vi "Process.vi"(0 "reg.notify host.go rcvd":bool, 1 "reg.reset":bool, 2 "reg.instruction fifo":refnum<k21>, 5 "reg.host read.go rcvd":bool, 7 "clock cross resources":T7, 9 "config.resources":T5, 11 "sync.resources":T6, 12 "time.resources":T3) -> (4 "reg.notify host.go":bool, 6 "reg.host read.data":T4)   [LabVIEW 2021]
doc: "The main process loop which sends instructions received from the host to its attached registers and returns register reads back to the host."
uses:
  Clock Cross Resources.ctl
  <instrlib>/niUsrpRio/Synchronization/v1/FPGA/Private/Resources.ctl
  <instrlib>/_niInstr/Register Bus/v1/FPGA/Public/Read Cmd Data.ctl
  <instrlib>/niUsrpRio/Time/v1/FPGA/Private/Time Resources.ctl
  <instrlib>/niUsrpRio/Time/v1/FPGA/Private/Future Event Resources.ctl
  <instrlib>/_niInstr/Register Bus/v1/FPGA/Public/Read Completion.ctl
  <instrlib>/_niInstr/Register Bus/v1/FPGA/Private/Mux/Read Completion Mux (2 inputs).vi
  <instrlib>/_niInstr/Register Bus/v1/FPGA/niInstr Register Bus v1 FPGA.lvlib
  <instrlib>/niUsrpRio/Synchronization/v1/FPGA/niUsrpRio Synchronization v1 FPGA.lvlib
  <instrlib>/niUsrpRio/Time/v1/FPGA/niUsrpRio Time v1 FPGA.lvlib
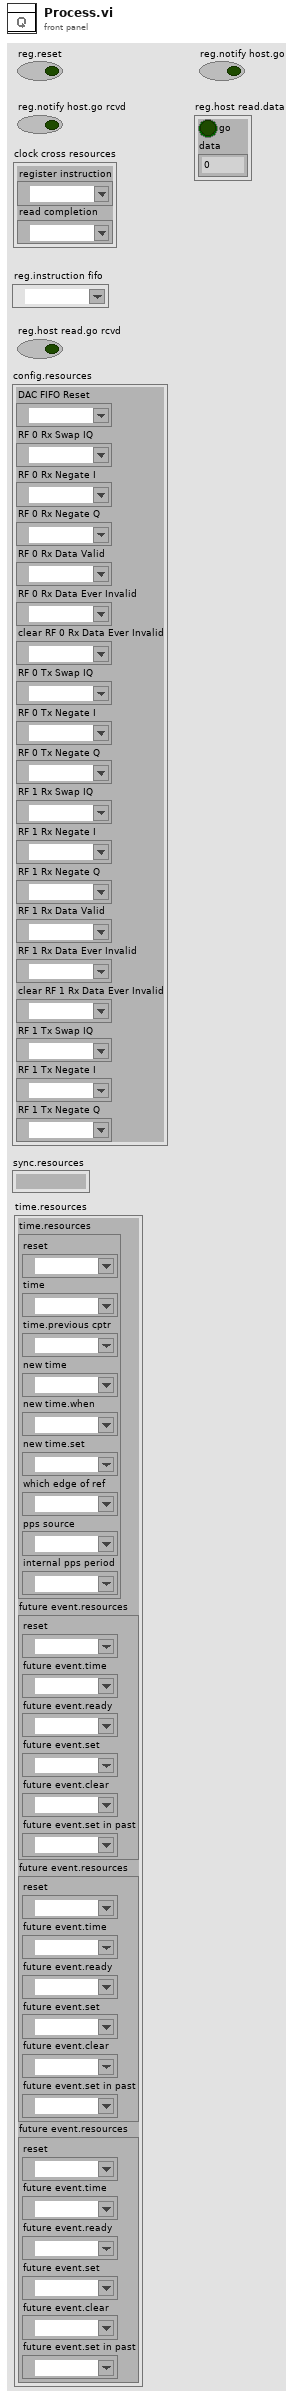
[diagram p1: front panel]
types:
  T1 = typedef "niUsrpRio Time v1 FPGA.lvlib/Time Resources.ctl" = cluster{"reset":refnum<k21>, "time":refnum<k21>, "time.previous cptr":refnum<k21>, "new time":refnum<k21>, "new time.when":refnum<k21>, "new time.set":refnum<k21>, "which edge of ref":refnum<k21>, "pps source":refnum<k21>, "internal pps period":refnum<k21>}
  T2 = typedef "niUsrpRio Time v1 FPGA.lvlib/Future Event Resources.ctl" = cluster{"reset":refnum<k21>, "future event.time":refnum<k21>, "future event.ready":refnum<k21>, "future event.set":refnum<k21>, "future event.clear":refnum<k21>, "future event.set in past":refnum<k21>}
  T3 = cluster{"time.resources":T1, "future event.resources":T2, "future event.resources":T2, "future event.resources":T2}
  T4 = typedef "niInstr Register Bus v1 FPGA.lvlib/Read Cmd Data.ctl" = cluster{"go":bool, "data":u32}
  T5 = cluster{"DAC FIFO Reset":refnum<k21>, "RF 0 Rx Swap IQ":refnum<k21>, "RF 0 Rx Negate I":refnum<k21>, "RF 0 Rx Negate Q":refnum<k21>, "RF 0 Rx Data Valid":refnum<k21>, "RF 0 Rx Data Ever Invalid":refnum<k21>, "clear RF 0 Rx Data Ever Invalid":refnum<k21>, "RF 0 Tx Swap IQ":refnum<k21>, "RF 0 Tx Negate I":refnum<k21>, "RF 0 Tx Negate Q":refnum<k21>, "RF 1 Rx Swap IQ":refnum<k21>, "RF 1 Rx Negate I":refnum<k21>, "RF 1 Rx Negate Q":refnum<k21>, "RF 1 Rx Data Valid":refnum<k21>, "RF 1 Rx Data Ever Invalid":refnum<k21>, "clear RF 1 Rx Data Ever Invalid":refnum<k21>, "RF 1 Tx Swap IQ":refnum<k21>, "RF 1 Tx Negate I":refnum<k21>, "RF 1 Tx Negate Q":refnum<k21>}
  T6 = typedef "niUsrpRio Synchronization v1 FPGA.lvlib/Resources.ctl" = cluster{"master":refnum<k21>, "meas.enable":refnum<k21>, "meas.ready":refnum<k21>, "meas.reset":refnum<k21>, "meas.arm":refnum<k21>, "meas.valid":refnum<k21>, "meas.value":refnum<k21>, "meas.oversample factor":refnum<k21>, "cptr":refnum<k21>, "cptr.adjust":refnum<k21>, "cptr.period":refnum<k21>}
  T7 = typedef "Clock Cross Resources.ctl" = cluster{"register instruction":refnum<k21>, "read completion":refnum<k21>}
  T8 = typedef "niInstr Register Bus v1 FPGA.lvlib/Read Completion.ctl" = cluster{"data":u32, "valid":bool}
  T9 = typedef "niInstr Register Bus v1 FPGA.lvlib/Register Instruction.ctl" = cluster{"subsystem":u8, "address":u16, "data":u32, "valid":bool, "read":bool}
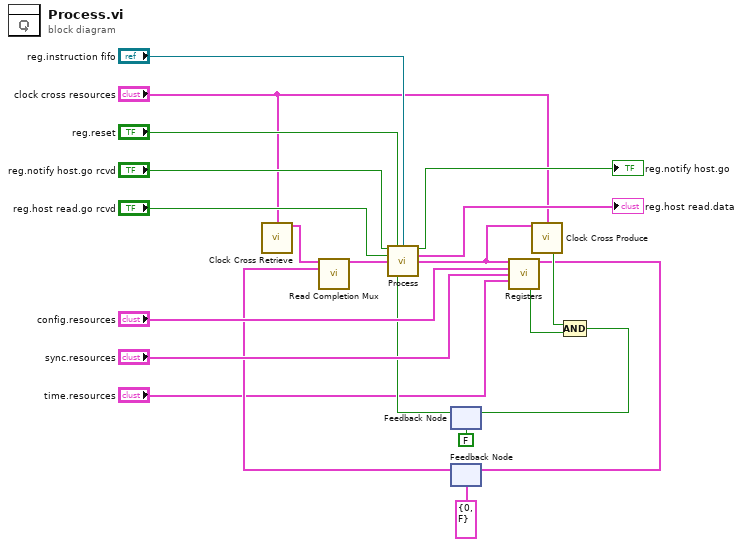
[diagram p0: block diagram]
diagram:
  n1 = call "Clock Cross Retrieve.vi"("resources"="clock cross resources") -> ("read completion out"=w2:T8)  [unwired: 14 in]
  n2 = feedback #1(FALSE) -> (w6:bool)
  n3 = feedback #2(T8 {"data"=0, "valid"=FALSE} ("read completion out")) -> (w3:T8)
  n4 = call-poly <instrlib>:"Read Completion Mux.vi"("element 0"=w2, "element 1"=w3) -> ("read completion out"=w21:T8)  [unwired: 13 in]
  n5 = call <instrlib>:"Process.vi"("reg.notify host.go rcvd"="reg.notify host.go rcvd", "reg.reset"="reg.reset", "reg.host instruction fifo"="reg.instruction fifo", "reg.host read.go rcvd"="reg.host read.go rcvd", "read completion"=w21, "ready for output"=w6) -> ("reg.notify host.go"=→"reg.notify host.go":bool, "reg.host read.data"=→"reg.host read.data":T4, "register instruction"=w10:T9)  [unwired: 7 in]
  n6 = call "Registers.vi"("register instruction"=w10, "config.resources"="config.resources", "sync.resources"="sync.resources", "time.resources"="time.resources") -> ("read completion out"=w8:T8, "ready for input"=w17:bool)  [unwired: 10 in]
  n7 = feedback-in #2(w8) -> ()
  n8 = call "Clock Cross Produce.vi"("register instruction"=w10, "resources"="clock cross resources") -> ("ready for input"=w9:bool)  [unwired: 13 in]
  n9 = Compound Arithmetic op=AND(w9, w17) -> (w7:bool)
  n10 = feedback-in #1(w7) -> ()
